vi "Get MCP Gain Table.vi"(8 "error in (no error)":errorcluster, 9 "pfPhotoepc":sgl, 10 "piGain":i32, 11 "iNum":i32) -> (0 "error out":errorcluster, 1 "pfPhotoepc out":sgl, 2 "piGain out":i32, 3 "function return":u32)   [LabVIEW 2014, in "atmcd32d.lvlib"]
doc: "unsigned int WINAPI GetMCPGainTable(int iNum, int * piGain, float * pfPhotoepc);"
uses:
  atmcd32d.lvlib
  atmcd32d.dll
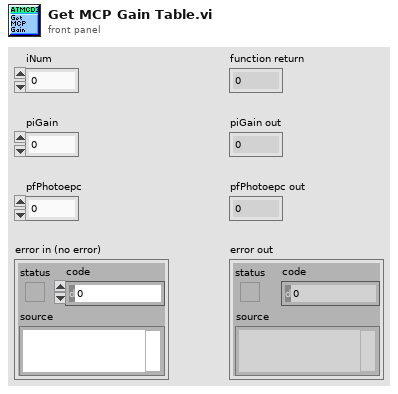
[diagram p1: front panel]
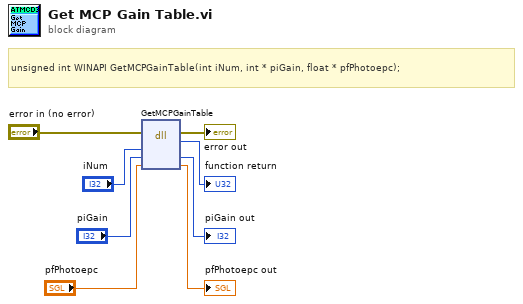
[diagram p0: block diagram]
diagram:
  # "unsigned int WINAPI GetMCPGainTable(int iNum, int * piGain, float * pfPhotoepc);"
  n1 = dll-call lib="C:/Users/Bakir/Documents/Lambda2-Testing/lib/Andorlib/atmcd32d.*" fn="GetMCPGainTable"(error in="error in (no error)", "iNum"="iNum", "piGain"="piGain", "pfPhotoepc"="pfPhotoepc") -> (error out=→"error out":errorcluster, →"function return":u32, "piGain"=→"piGain out":i32, "pfPhotoepc"=→"pfPhotoepc out":sgl)  [unwired: 3 in, 1 out]
